vi "401_Export_ Report_Html.vi"(0 "Enum":enum16{"HTML", "PDF"}(ring), 2 "Data":string[][](array[string])=[["1", "A", "2313213", "fsdgdsfgsdfg"], ["2", "B", "fgndfb", "dfgdfgdfg"], ["3", "C", "dfgdfg", "dfgdfgdfg"]], 3 "column headers":string[](array[string])=["S.NO", "User Name", "Date Timne", "Activity"]) -> (19 "Error out":errorcluster)   [LabVIEW 2015]
uses:
  <vilib>/Utility/NIReport.llb/HTML Report Text Alignment.ctl
  System Settings/Modules/LV2GActions.ctl
  <vilib>/Utility/NIReport.llb/Append Text Table to Report (wrap).vi
  <vilib>/Utility/NIReport.llb/Append Report Text (str wrap).vi
  <vilib>/Utility/NIReport.llb/NI_report.lvclass
  <vilib>/Utility/NIReport.llb/NI_ReportGenerationCore.lvlib
  <vilib>/Platform/browser.llb/Open URL in Default Browser (string).vi
panel:
  out "Error out 2":errorcluster
  out "error out 2":errorcluster
  in  "error in (no error)":errorcluster
  in  "Total":dbl[](array[numeric])
  in  "Fail":dbl[](array[numeric])
  in  "Plot names":string[](array[string])
  in  "Array":dbl[](array[numeric])
  # "Input"
  # "Output"
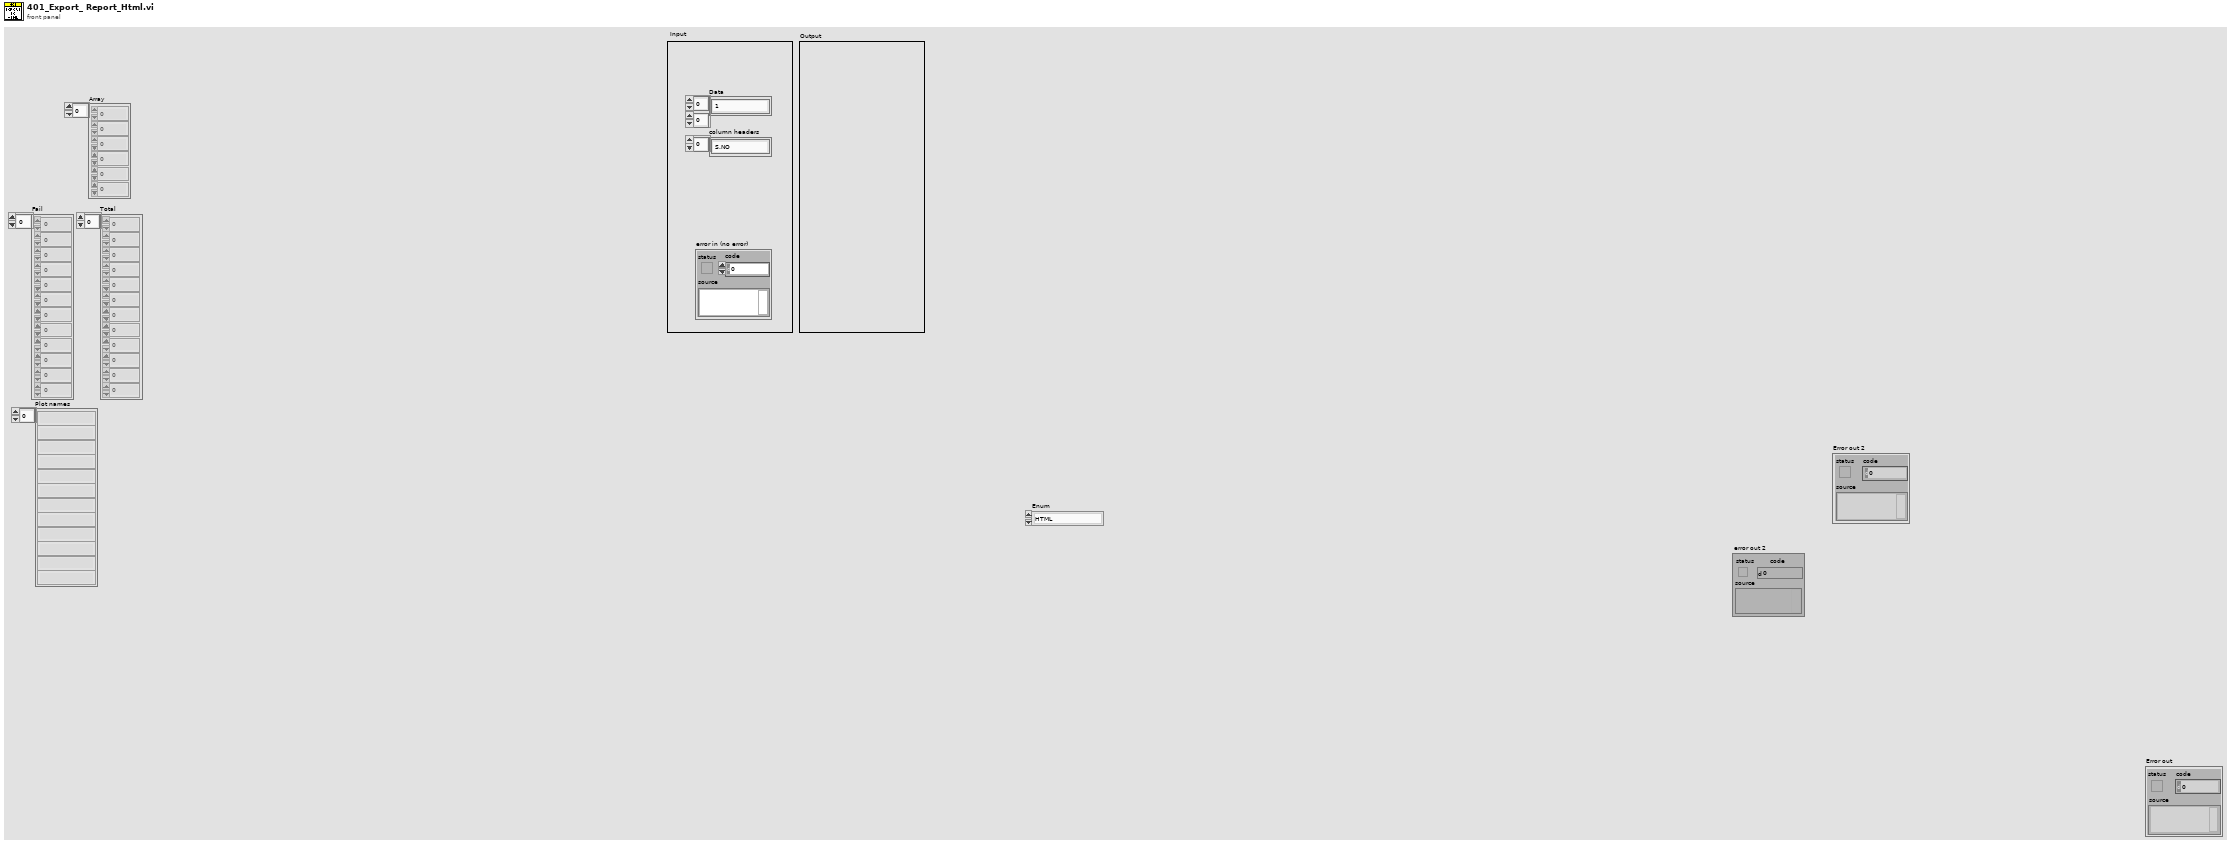
[diagram p1: front panel]
types:
  T1 = typedef "LV2GActions.ctl" = enum16{"Read", "Write", "Current", "Update", "UpdateSystemSettings", "UpdateModel"}
  T2 = enum16{"Read", "Current", "UpdateRecipiePath", "UpdateBatchPath"}
  T3 = typedef "NI_ReportGenerationCore.lvlib/HTML Report Text Alignment.ctl" = enum16{"(default)", "LEFT", "CENTER", "RIGHT"}
  T4 = enum16{"maximized", "minimized", "normal", "no change"}
  T5 = enum16{"Standard Report", "HTML", "Word", "Excel"}
  T6 = cluster{"BasePath":path, "RecipiePath":path, "BatchPath":path}
  T7 = cluster{"UserName":string, "Group Level":u16, "Theme":u16, "Software Type":u16, "System Language":u16, "Master":bool, "Recipe":string, "Batch":string, "Simulate":bool, "Trigger Activation":u16, "DateFormat":u16, "HardwareTest":bool}
  T8 = typedef "401_Productionsettings.ctl" = cluster{"Company Name":string, "Machine ID":string, "Empty":bool, "Missing":bool, "Size":bool, "Spot":bool, "Color":bool, "Foreign Particle":bool, "Different Particles":bool, "Product Foil":bool}
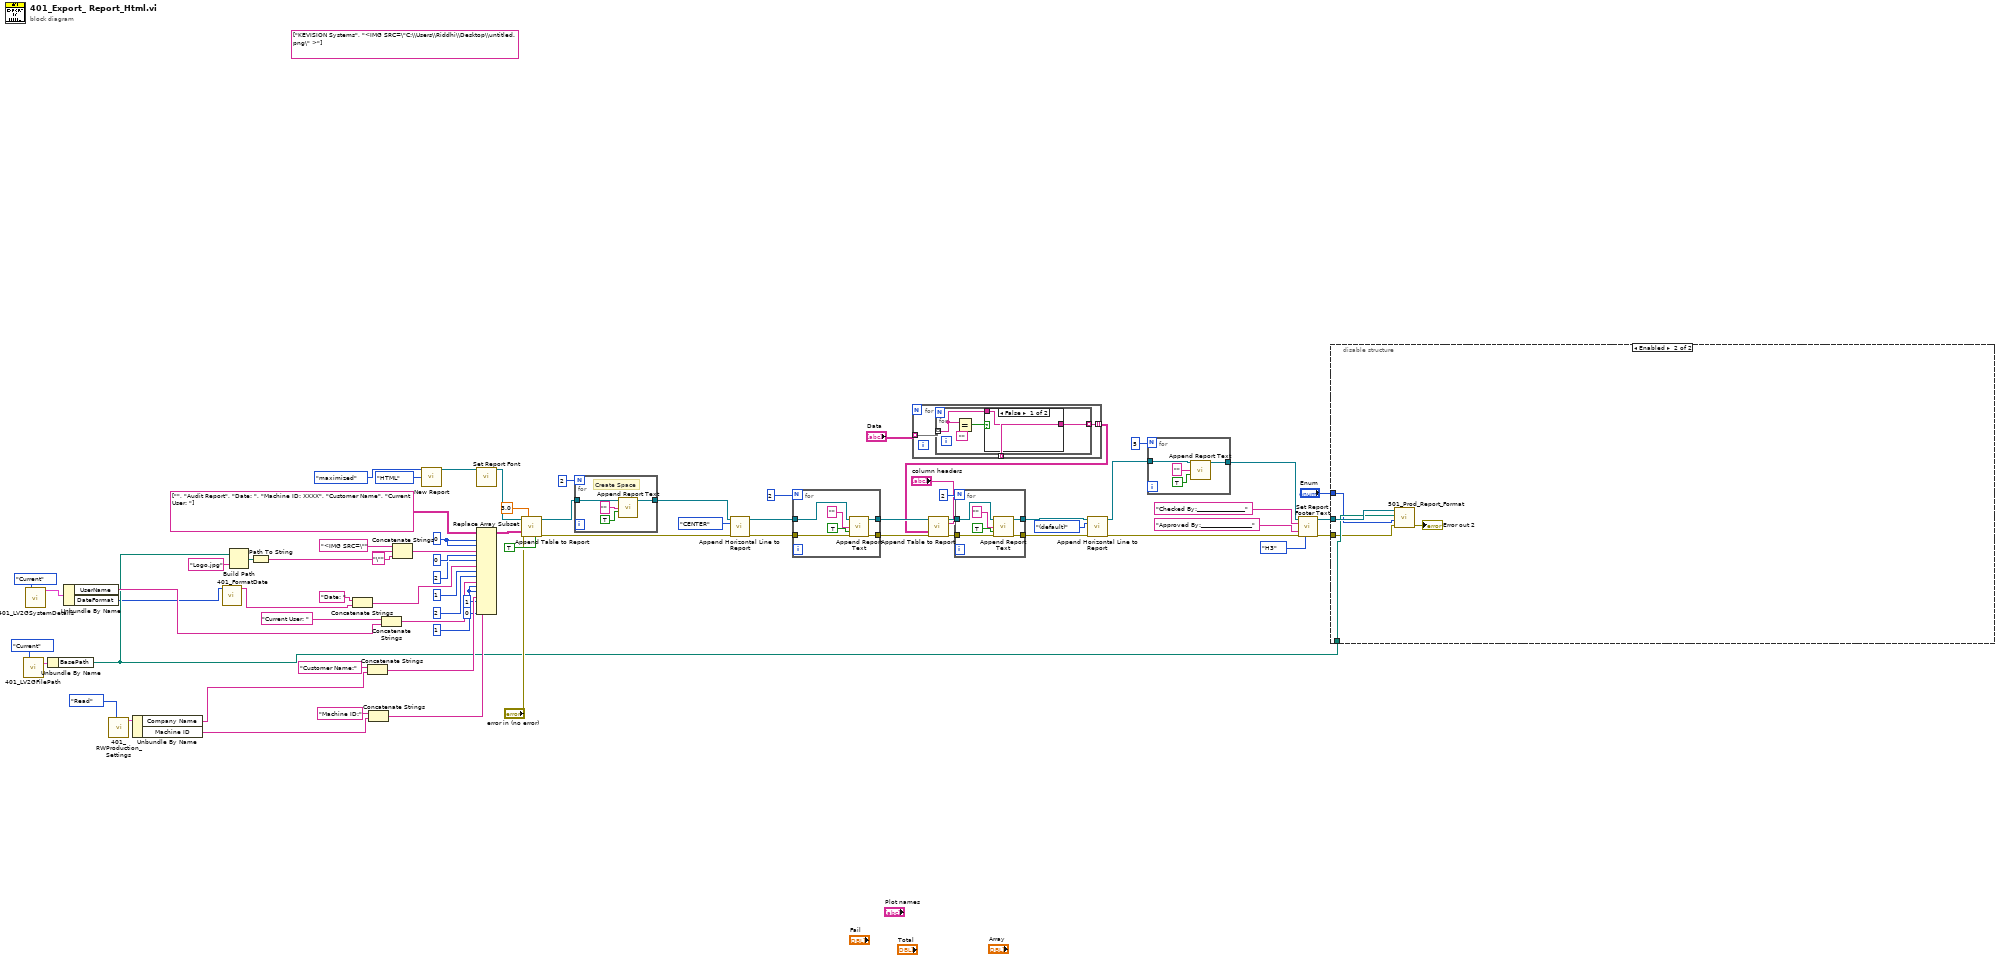
[diagram p0: block diagram]
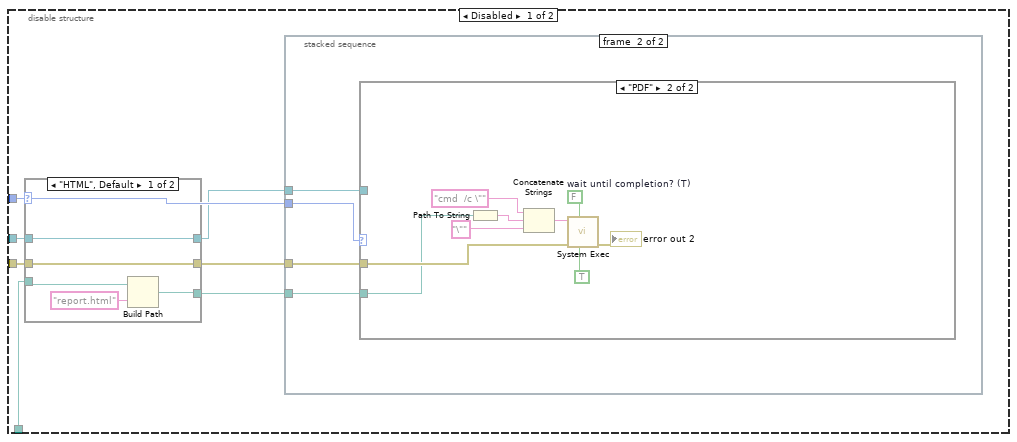
[diagram p2: hidden frame]
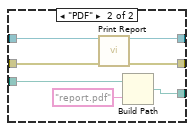
[diagram p3: hidden frame]
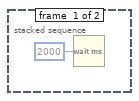
[diagram p4: hidden frame]
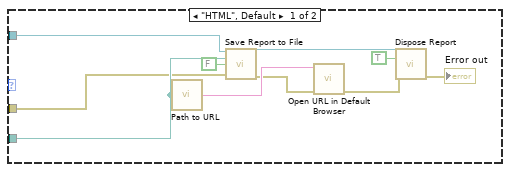
[diagram p5: hidden frame]
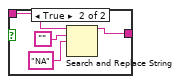
[diagram p6: hidden frame]
diagram:
  w62 = 1 ("index (row)")
  w67 = 0 ("index (row)")
  (unwired) string[] ["KEVISION Systems", "<IMG SRC=\"C:\\Users\\Riddhi\\Desktop\\untitled.png\" >"] ("text data")
  n1 = call "401_LV2GFilePath.vi"("Read"=T2."Current") -> ("Path"=w27:T6)  [unwired: 17 in, 1 out]
  n2 = call "401_LV2GSystemDetails.vi"("R/W/C"=LV2GActions."Current") -> ("DataOut"=w26:T7)  [unwired: 17 in, 1 out]
  n3 = Unbundle By Name(w27) -> ("BasePath"=w3:path)
  n4 = Unbundle By Name(w26) -> ("UserName"=w25:string, "DateFormat"=w2:u16)
  n5 = call "401_RWProduction_Settings.vi"("Action"=enum16{"Read", "Write"}."Read") -> ("Data Out"=w13:T8)  [unwired: 9 in, 1 out]
  n6 = Unbundle By Name(w13) -> ("Company Name"=w12:string, "Machine ID"=w8:string)
  n7 = call "401_FormatDate.vi"("DateFormat"=w2) -> ("date/time string"=w1:string)  [unwired: 10 in]
  n8 = Build Path(base path=w3, name or relative path="Logo.jpg") -> (appended path=w23:path)
  n9 = Path To String(path=w23) -> (string=w22:string)
  n10 = Concatenate Strings("Date: " ("string"), w1) -> (w53:string)
  n11 = Concatenate Strings("Customer Name:" ("string"), w12) -> (w16:string)
  n12 = Concatenate Strings("Machine ID:" ("string"), w8) -> (w7:string)
  n13 = Concatenate Strings("Current User: " ("string"), w25) -> (w52:string)
  n14 = Concatenate Strings("<IMG SRC=\"" ("string"), w22, "\"" ("string")) -> (w59:string)
  n15 = call <vilib>:"New Report.vi"("window state (normal)"=T4."maximized", "report type"=T5."HTML") -> ("report out"=w70:refnum<class "NI_report.lvclass">)  [unwired: 12 in, 1 out]
  n16 = call-dynamic "Set Report Font.vi"("report in"=w70) -> ("report out"=w57:refnum<class "NI_report.lvclass">)  [unwired: 12 in, 2 out]
  n17 = Replace Array Subset(array=string[][] [["", "Audit Report", "Date: "], ["Machine ID: XXXX", "Customer Name", "Current User: "]] ("text data"), new element #1=w59, index (row) #1=w67, index (col) #1=w67, new element #2=w53, index (row) #2=0 ("index (row)"), index (col) #2=2 ("disabled index (col)"), new element #3=w52, index (row) #3=1 ("index (row)"), index (col) #3=2 ("disabled index (col)"), new element #4=w16, index (row) #4=w62, index (col) #4=w62, new element #5=w7, index (row) #5=1 ("index (row)"), index (col) #5=0 ("disabled index (col)")) -> (w68:string[][])
  n18 = call-poly <vilib>:"Append Table to Report.vi"("report in"=w57, "column width (1)"=3.0, "text data"=w68, "error in (no error)"="error in (no error)", "show grid lines (YES)"=TRUE) -> ("report out"=w47:refnum<class "NI_report.lvclass">, "error out"=w51:errorcluster)  [unwired: 7 in, 2 out]
  n19 = for {
    N: 2 -> [_]
    tunnel: w47 -> [w74]
    tunnel: [w73] -> w46
    # "Create Space"
    n20 = call-poly <vilib>:"Append Report Text.vi"("report in"=w74, "text"="", "append on new line? (F)"=TRUE) -> ("report out"=w73:refnum<class "NI_report.lvclass">)  [unwired: 9 in, 3 out]
  }
  n21 = call-dynamic "Append Horizontal Line to Report.vi"("report in"=w46, "align (default)"=HTML_Report_Text_Alignment."CENTER", "error in (no error)"=w51) -> ("report out"=w41:refnum<class "NI_report.lvclass">, "error out"=w40:errorcluster)  [unwired: 11 in]
  n22 = for {
    N: 2 -> [_]
    tunnel: w41 -> [w80]
    tunnel: [w79] -> w38
    tunnel: w40 -> [w78]
    tunnel: [w77] -> w39
    n23 = call-poly <vilib>:"Append Report Text.vi"("report in"=w80, "text"="", "append on new line? (F)"=TRUE, "error in (no error)"=w78) -> ("report out"=w79:refnum<class "NI_report.lvclass">, "error out"=w77:errorcluster)  [unwired: 8 in, 2 out]
  }
  n24 = for {
    tunnel: "Data" -> [w84] mode=indexing
    tunnel: [w83] -> w17 mode=indexing
    tunnel: [w83] -> _ mode=indexing
    n25 = for {
      tunnel: w84 -> [w85] mode=indexing
      tunnel: [w88] -> w83 mode=indexing
      n26 = Equal?(x=w85, y="") -> (x = y?=w87:bool)
      n27 = case shown="False" w87 {
        tunnel: w85 -> [w89 w93]
        tunnel: [w89 w90] -> w88
        frame False {
        }
        frame True {
          n28 = Search and Replace String(input string=w93, search string="", replace string="NA" ("replace string (\"\")")) -> (result string=w90:string)  [unwired: 5 in, 3 out]
        }
      }
    }
  }
  n29 = call-poly <vilib>:"Append Table to Report.vi"("report in"=w38, "column headers"="column headers", "text data"=w17, "error in (no error)"=w39) -> ("report out"=w33:refnum<class "NI_report.lvclass">, "error out"=w34:errorcluster)  [unwired: 8 in, 2 out]
  n30 = for {
    N: 2 -> [_]
    tunnel: w33 -> [w97]
    tunnel: [w96] -> w31
    tunnel: w34 -> [w95]
    tunnel: [w94] -> w30
    n31 = call-poly <vilib>:"Append Report Text.vi"("report in"=w97, "text"="", "append on new line? (F)"=TRUE, "error in (no error)"=w95) -> ("report out"=w96:refnum<class "NI_report.lvclass">, "error out"=w94:errorcluster)  [unwired: 8 in, 2 out]
  }
  n32 = call-dynamic "Append Horizontal Line to Report.vi"("report in"=w31, "align (default)"=HTML_Report_Text_Alignment."(default)", "error in (no error)"=w30) -> ("report out"=w21:refnum<class "NI_report.lvclass">, "error out"=w44:errorcluster)  [unwired: 11 in]
  n33 = for {
    N: 5 -> [_]
    tunnel: [w101] -> w42
    tunnel: w21 -> [w100]
    n34 = call-poly <vilib>:"Append Report Text.vi"("report in"=w100, "text"="", "append on new line? (F)"=TRUE) -> ("report out"=w101:refnum<class "NI_report.lvclass">)  [unwired: 9 in, 3 out]
  }
  n35 = call-dynamic "Set Report Footer Text.vi"("report in"=w42, "left footer text"="Checked By:________________" ("text"), "right footer text"="Approved By:_________________", "error in (no error)"=w44, "HTML footer size"=enum16{"H1", "H2", "H3", "H4", "H5", "H6", "H7"}."H3") -> ("report out"=w6:refnum<class "NI_report.lvclass">, "error out"=w5:errorcluster)  [unwired: 9 in]
  n36 = disable-structure shown="Enabled" {
    disable-tunnel: w6 -> [w110 w151]
    disable-tunnel: w5 -> [w109 w149]
    disable-tunnel: "Enum" -> [w107 w147]
    disable-tunnel: w3 -> [w105 w150]
    frame Disabled {
      n37 = case shown="\"HTML\", Default" w107 {
        tunnel: w110 -> [w114 w122]
        tunnel: w109 -> [w115 w121]
        tunnel: [w115 w120] -> w108
        tunnel: [w114 w119] -> w106
        tunnel: w105 -> [w112 w117]
        tunnel: [w111 w116] -> w104
        frame "HTML", Default {
          n38 = Build Path(base path=w112, name or relative path="report.html") -> (appended path=w111:path)
        }
        frame "PDF" {
          n39 = call-dynamic "Print Report.vi"("report in"=w122, "error in (no error)"=w121) -> ("report out"=w119:refnum<class "NI_report.lvclass">, "error out"=w120:errorcluster)  [unwired: 12 in]
          n40 = Build Path(base path=w117, name or relative path="report.pdf") -> (appended path=w116:path)
        }
      }
      n41 = stacked-sequence {
        tunnel: w108 -> [_ w127]
        tunnel: w107 -> [_ w126]
        tunnel: w106 -> [_ w125]
        tunnel: w104 -> [_ w124]
        frame #0 {
          n42 = Wait (ms)(milliseconds to wait=u32 2000) -> ()  [unwired: 1 out]
        }
        frame #1 {
          n43 = case shown="\"PDF\"" w126 {
            tunnel: w127 -> [w129 w139]
            tunnel: w124 -> [w130 w138]
            tunnel: w125 -> [w128 _]
            frame "HTML", Default {
              n44 = call <vilib>:"Path to URL.vi"("path"=w130) -> ("url"=w133:string)
              n45 = call-dynamic "Save Report to File.vi"("report in"=w128, "report file path"=w130, "prompt to replace? (F)"=FALSE, "error in (no error)"=w129) -> ("report out"=w134:refnum<class "NI_report.lvclass">, "error out"=w132:errorcluster)  [unwired: 10 in]
              n46 = call-poly <vilib>:"Open URL in Default Browser.vi"("error in (no error)"=w132, "URL"=w133) -> ("error out"=w137:errorcluster)  [unwired: 4 in, 1 out]
              n47 = call-dynamic "Dispose Report.vi"("report in"=w134, "wait until printing completed? (T)"=TRUE, "error in (no error)"=w137) -> ("error out"=→"Error out":errorcluster)  [unwired: 12 in]
            }
            frame "PDF" {
              w146 = FALSE  # wait until completion? (T)
              n48 = Path To String(path=w138) -> (string=w142:string)
              n49 = Concatenate Strings("cmd  /c \"", w142, "\"") -> (w144:string)
              n50 = call <vilib>:"System Exec.vi"("run minimized? (F)"=TRUE, "wait until completion? (T)"=w146, "error in (no error)"=w139, "command line"=w144) -> ("error out"=→"error out 2":errorcluster)  [unwired: 4 in, 3 out]
            }
          }
        }
      }
    }
    frame Enabled {
      n51 = call "501_Prod_Report_Format.vi"("error in (no error)"=w149, "Enum"=w147, "BasePath"=w150, "NI_report in"=w151) -> ("Error out"=→"Error out 2":errorcluster)  [unwired: 7 in]
    }
  }
